vi "Climb Loop.vi"(10 "Extend Power in":dbl, 11 "Y Power":dbl) -> (1 "Unpin?":bool, 2 "Pull Power":dbl, 3 "PTO Engaged?":bool, 5 "Extend Power":dbl)   [LabVIEW 2015]
uses:
  Robot Global Data.vi
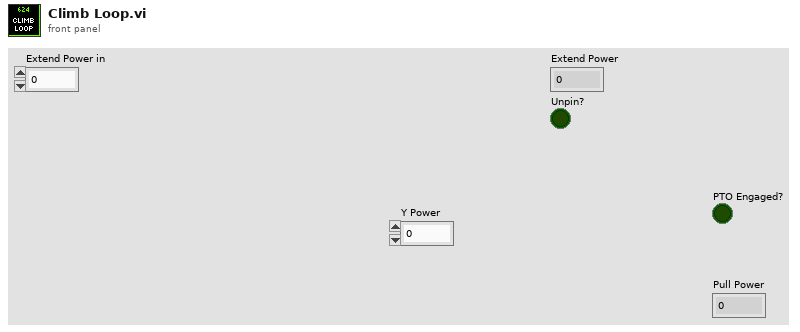
[diagram p1: front panel]
types:
  T1 = typedef "Dashboard Control Data.ctl" = cluster{"Encoder Control":T2, "Steer PID output":cluster{"output high":dbl, "output low":dbl}, " Steer PID gains":cluster{"proportional gain (Kc)":dbl, "integral time (Ti, min)":dbl, "derivative time (Td, min)":dbl}, "Drivetrain Settings":T3, "Vision Packet":T4, "Dashboard Drivetrain Command":T5, "Info/Command Cluster":T7, "Ball Vision Packet":T8, "Intake Presets":T10, "Intake Encoder Control":T12, "Climb Presets":T13, "Goal Output Range":cluster{"output high":dbl, "output low":dbl}, "Enabled Systems":T14, "Auton Presets":T15, "Pressure M":dbl, "Pressure B":dbl, "Vision Timeout":dbl, "Auto-Shift":T16, "Catapult Setpoints":T17}
  T2 = typedef "Encoder Control.ctl" = cluster{"Right Tick Constant":dbl, "Left Tick Constant":dbl, "Reset?":bool, "Y Dist":cluster{"PID gains":cluster{"proportional gain (Kc)":dbl, "integral time (Ti, min)":dbl, "derivative time (Td, min)":dbl}}, "Y Stop Thresh":dbl, "Y Stop Speed":dbl}
  T3 = typedef "Drivetrain Settings.ctl" = cluster{"Gyro Tolerance":dbl, "Throttle Ramp (ms)":dbl, "Kv":dbl, "Ka":dbl, "Feed Forward P":dbl, "Feed Forward D":dbl, "Goal Vision PID gains":cluster{"proportional gain (Kc)":dbl, "integral time (Ti, min)":dbl, "derivative time (Td, min)":dbl}, "Goal Detection Window":dbl, "Creep Rate":dbl, "Vision Throttle Threshold":dbl, "Min Turn Output":dbl, "Left Batter Angle":dbl, "Right Batter Angle":dbl}
  T4 = typedef "Goal Vision Packet.ctl" = cluster{"Distance":dbl, "Center X":dbl, "Center Y":dbl, "Found Target?":bool, "Robot Center":dbl, "Angle":dbl}
  T5 = typedef "Dashboard Drivetrain Command.ctl" = cluster{"Drivetrain Vision":T6}
  T6 = typedef "Drivetrain Vision.ctl" = cluster{"Goal Window":dbl, "Ball Window":dbl}
  T7 = typedef "Ball Tracking Command Cluster.ctl" = cluster{"Distance to Ball":dbl, "Desired Angle":dbl, "Command":enum16{"Turn to Ball", "Turn to Angle", "Get Distance"}, "Pixels from Center":dbl}
  T8 = typedef "Ball Vision Packet.ctl" = cluster{"Ball Detected?":bool, "Distance to Ball":dbl, "Desired Angle":dbl, "Pixels from Center":dbl, "Tracking mode":T9}
  T9 = typedef "Tracking Mode.ctl" = enum16{"Turn to Ball", "Turn to Angle"}
  T10 = typedef "Intake Presets.ctl" = cluster{"Intake Speed":dbl, "Outake Speed":dbl, "Low Height":dbl, "Half Height":dbl, "High Idle Height":dbl, "Angle Speed":dbl, "Angle Tolerance":dbl, "Encoder Scale":dbl, "Load Height":dbl, "Output Range":T11, "Rotation Power Max/Min":dbl, "MaxCurrent":dbl, "Intake Trip Time":dbl, "Idle Height":dbl, "Max Height":dbl, "Reset Encoders?":bool, "PID gains":cluster{"proportional gain (Kc)":dbl, "integral time (Ti, min)":dbl, "derivative time (Td, min)":dbl}, "Intake Stop Delay":u32, "Settle Time":dbl, "Settle Wait Time":dbl, "Pull Up Delay":dbl}
  T11 = typedef "Drivetrain Output Range.ctl" = cluster{"output high":dbl, "output low":dbl}
  T12 = typedef "IntakeEcoderControl.ctl" = cluster{"Arm Tick Constant":dbl, "Reset?":bool, "Y Dist":cluster{"PID gains":cluster{"proportional gain (Kc)":dbl, "integral time (Ti, min)":dbl, "derivative time (Td, min)":dbl}}, "Y Stop Thresh":dbl, "Y Stop Speed":dbl}
  T13 = typedef "Climb Presets.ctl" = cluster{"Pull Power":dbl, "Extend Power":dbl}
  T14 = typedef "Enabled Systems.ctl" = cluster{"Shoot":bool, "Intake":bool, "DT":bool, "Gyro":bool, "100ms":bool, "US":bool}
  T15 = typedef "Autonomous Presets.ctl" = cluster{"Pitch Limit":dbl, "Roll Limit":dbl, "Start Position":dbl, "Cross Position":dbl}
  T16 = typedef "Auto Shift Cluster.ctl" = cluster{"Delay":dbl, "Speed Thresh":dbl, "Upshift Accel":dbl, "Upshift Throttle":dbl, "Upshift Throttle Accel":dbl, "Downshift Throttle":dbl, "Downshift Throttle Accel":dbl, "Pressure Threshold":dbl}
  T17 = typedef "Catapult Presets.ctl" = cluster{"Intake Danger Height":dbl, "Ball Security Delay ":dbl, "High PSI Minimum":dbl, "Shot Finish Delay":dbl, "Low PSI Minimum":dbl, "Idle Ball Security Wait ":dbl}
  T18 = typedef "Climb Command Cluster.ctl" = cluster{"Climb Mode":T19, "Hold?":bool, "Manual State":T20}
  T19 = typedef "Climb Mode.ctl" = enum16{"Auto", "Semi-Auto", "Manual"}
  T20 = typedef "Climb Manual State.ctl" = cluster{"Release":bool, " PTO Engage":bool, "Extend":bool}
  T21 = typedef "Climb Status Cluster.ctl" = cluster{"Pull Power":dbl, "Unpin Power":dbl, "PTO Engaged?":bool, "Climb Mode":T19}
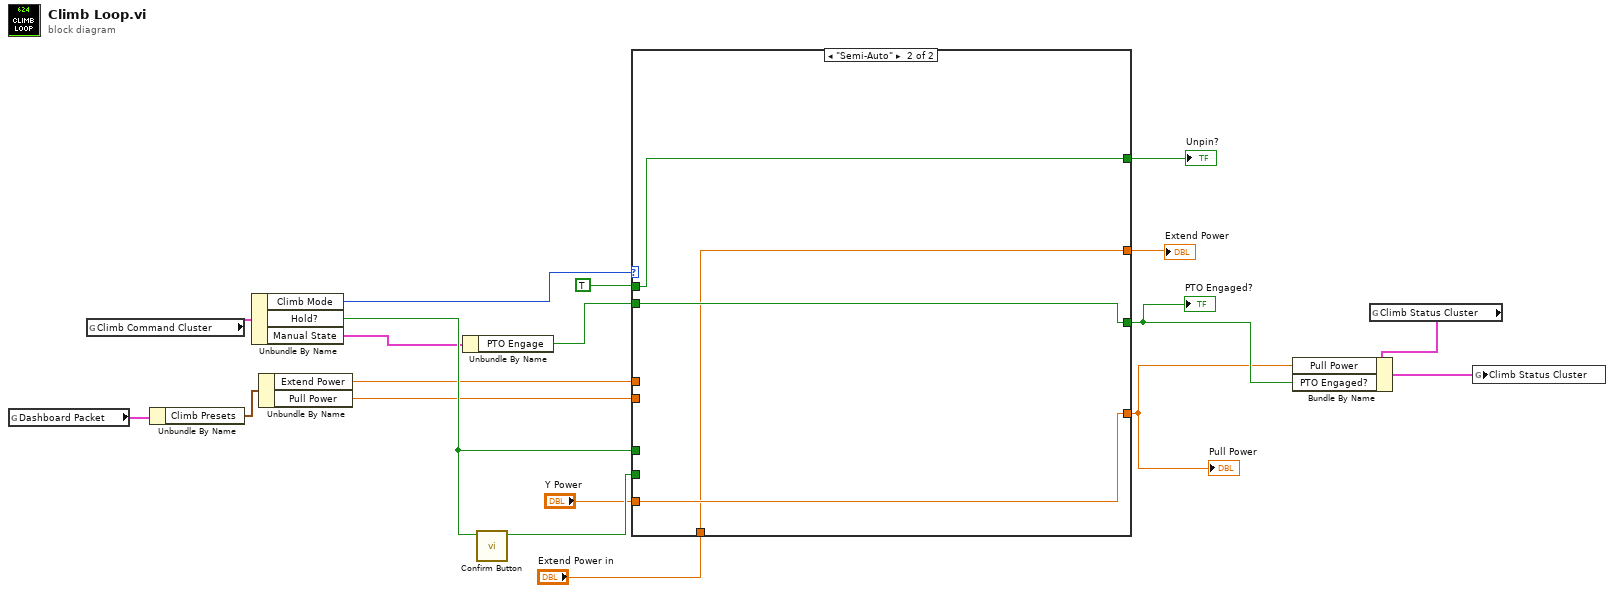
[diagram p0: block diagram]
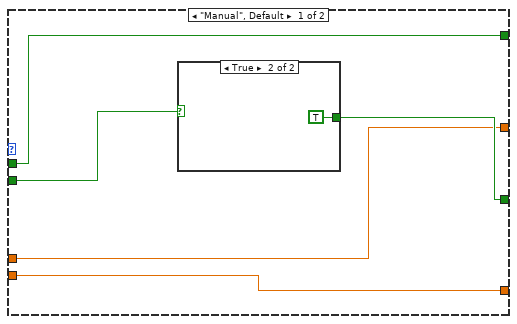
[diagram p2: hidden frame]
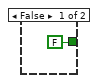
[diagram p3: hidden frame]
diagram:
  n1 = global read "Robot Global Data.vi" "Dashboard Packet"() -> (w15:T1)
  n2 = global read "Robot Global Data.vi" "Climb Command Cluster"() -> (w17:T18)
  n3 = Unbundle By Name(w15) -> ("Climb Presets"=w9:T13)
  n4 = Unbundle By Name(w17) -> ("Climb Mode"=w18:T19, "Hold?"=w16:bool, "Manual State"=w4:T20)
  n5 = Unbundle By Name(w9) -> ("Extend Power"=w11:dbl, "Pull Power"=w10:dbl)
  n6 = Unbundle By Name(w4) -> ("PTO Engage"=w5:bool)
  n7 = call "Confirm Button.vi"("Button"=w16) -> ("Boolean out"=w19:bool)  [unwired: 10 in]
  n8 = case shown="\"Semi-Auto\"" w18 {
    tunnel: w11 -> [w20 _]
    tunnel: [w21 w29] -> w13
    tunnel: [w22 w28] -> w14
    tunnel: TRUE ("Release") -> [w24 w30]
    tunnel: w19 -> [_ _]
    tunnel: w5 -> [w23 w28]
    tunnel: w10 -> [w21 _]
    tunnel: w16 -> [_ _]
    tunnel: [w24 w30] -> w12
    tunnel: [w20 w27] -> w6
    tunnel: "Y Power" -> [_ w29]
    tunnel: "Extend Power in" -> [_ w27]
    frame "Manual", Default {
      n9 = case shown="True" w23 {
        tunnel: [FALSE TRUE] -> w22
        frame False {
        }
        frame True {
        }
      }
    }
    frame "Semi-Auto" {
    }
  }
  "Pull Power" <- w13
  "PTO Engaged?" <- w14
  "Extend Power" <- w6
  "Unpin?" <- w12
  n10 = global read "Robot Global Data.vi" "Climb Status Cluster"() -> (w7:T21)
  n11 = Bundle By Name(cluster=w7, "Pull Power"=w13, "PTO Engaged?"=w14) -> (w8:T21)
  n12 = global write "Robot Global Data.vi" "Climb Status Cluster"(w8) -> ()
